vi "Self Configure.vi"(8 "error in (no error)":errorcluster, 11 "Instruments in":refnum<class "Instruments.lvclass">) -> (0 "error out":errorcluster, 3 "Instruments out":refnum<class "Instruments.lvclass">)   [LabVIEW 2023, in "Instruments.lvlib" / "Instruments.lvclass"]
uses:
  Library/Instruments.lvclass
  Custom Controls/Configuration Keys.ctl
  Library/Instruments.lvclass/Instruments.ctl
  builds/Framework/Configuration.lvlibp/Library/Configuration.lvclass
  C:/Users/Public/Documents/Development/builds/Framework/Configuration.lvlibp/Library/Configuration.lvclass
panel:
  in  "Configuration Keys":T1
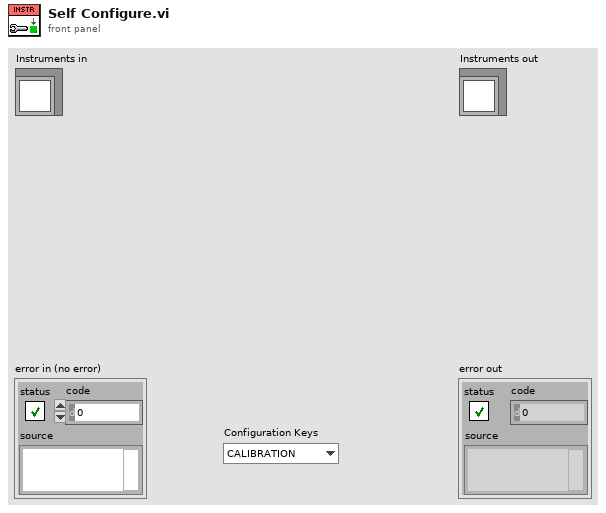
[diagram p1: front panel]
types:
  T1 = typedef "Instruments.lvlib/Instruments.lvclass/Configuration Keys.ctl" = enum16{"CALIBRATION", "RESOURCE", "POLL(MS)", "PANEL", "SIMULATED", "ENABLED"}
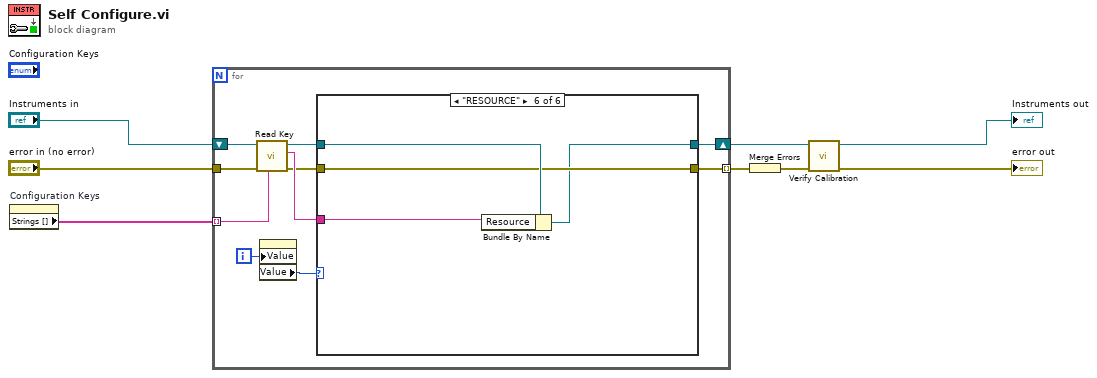
[diagram p0: block diagram]
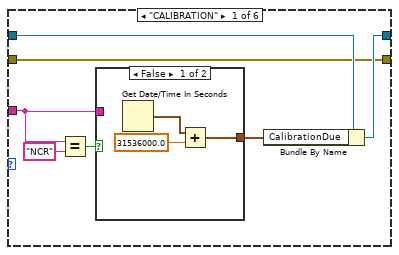
[diagram p2: hidden frame]
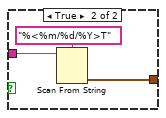
[diagram p3: hidden frame]
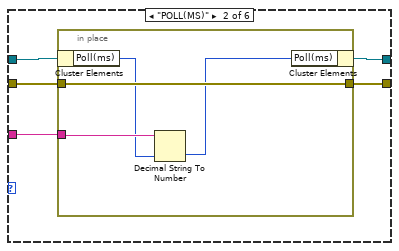
[diagram p4: hidden frame]
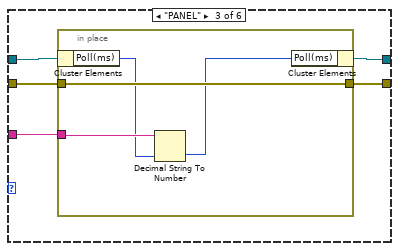
[diagram p5: hidden frame]
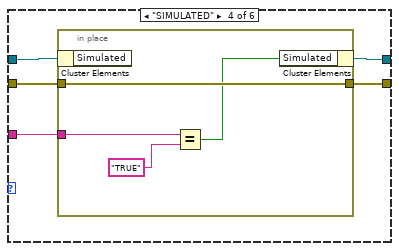
[diagram p6: hidden frame]
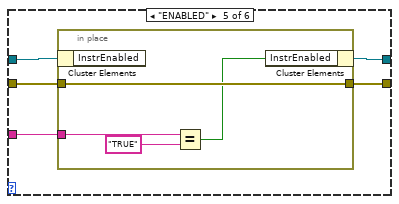
[diagram p7: hidden frame]
diagram:
  n1 = property on="Configuration Keys" class="Enum (strict)"() -> ("Strings []"=w7:string[])  [unwired: 2 in, 2 out]
  n2 = for {
    shift-right: [w10] -> w4
    shift-left: "Instruments in" -> [w16]
    tunnel: w7 -> [w13] mode=indexing
    tunnel: "error in (no error)" -> [w14]
    tunnel: [w9] -> w5 mode=indexing
    i -> [w18]
    n3 = call "Read Key.vi"("Key"=w13, "error in (no error)"=w14, "Configuration in"=w16) -> ("error out"=w11:errorcluster, "Value"=w12:string, "Configuration out"=w15:refnum<class "Instruments.lvclass">)  [unwired: 6 in]
    n4 = property on="Configuration Keys" class="Enum (strict)"("Value"=w18) -> ("Value"=w17:T1)  [unwired: 2 in, 2 out]
    n5 = case shown="\"RESOURCE\"" w17 {
      tunnel: w15 -> [w25 w36 w45 w54 w63 w71]
      tunnel: w12 -> [w19 w32 w41 w50 w59 w68]
      tunnel: w11 -> [w23 w34 w43 w52 w61 w70]
      tunnel: [w24 w35 w44 w53 w62 w69] -> w10
      tunnel: [w23 w33 w42 w51 w60 w70] -> w9
      frame "CALIBRATION" {
        n6 = Equal?(x=w19, y="NCR") -> (x = y?=w21:bool)
        n7 = case shown="False" w21 {
          tunnel: [w26 w29] -> w20
          tunnel: w19 -> [_ w31]
          frame False {
            n8 = Get Date/Time In Seconds() -> (seconds since 1Jan1904=w28:timestamp)
            n9 = Add(x=w28, y=31536000.0) -> (x+y=w26:timestamp)
          }
          frame True {
            n10 = Scan From String(format string="%<%m/%d/%Y>T", input string=w31) -> (output 1=w29:timestamp)  [unwired: 3 in, 3 out]
          }
        }
        n11 = Bundle By Name(cluster=w25, "CalibrationDue"=w20) -> (w24:refnum<class "Instruments.lvclass">)
      }
      frame "POLL(MS)" {
        n12 = in-place {
          in-place-border: w34 -> [w40]
          in-place-border: [w40] -> w33
          in-place-border: w32 -> [w39]
          n13 = in-place-cluster #1(w36) -> ("Poll(ms)"=w38:i32)
          n14 = Decimal String To Number(string=w39, default (0L)=w38) -> (number=w37:i32)  [unwired: 1 in, 1 out]
          n15 = in-place-cluster #1("Poll(ms)"=w37) -> (w35:refnum<class "Instruments.lvclass">)
        }
      }
      frame "PANEL" {
        n16 = in-place {
          in-place-border: w43 -> [w49]
          in-place-border: [w49] -> w42
          in-place-border: w41 -> [w48]
          n17 = in-place-cluster #2(w45) -> ("Poll(ms)"=w47:i32)
          n18 = Decimal String To Number(string=w48, default (0L)=w47) -> (number=w46:i32)  [unwired: 1 in, 1 out]
          n19 = in-place-cluster #2("Poll(ms)"=w46) -> (w44:refnum<class "Instruments.lvclass">)
        }
      }
      frame "SIMULATED" {
        n20 = in-place {
          in-place-border: w52 -> [w58]
          in-place-border: [w58] -> w51
          in-place-border: w50 -> [w57]
          n21 = in-place-cluster #3(w54) -> ()  [unwired: 1 out]
          n22 = Equal?(x=w57, y="TRUE") -> (x = y?=w55:bool)
          n23 = in-place-cluster #3("Simulated"=w55) -> (w53:refnum<class "Instruments.lvclass">)
        }
      }
      frame "ENABLED" {
        n24 = in-place {
          in-place-border: w61 -> [w67]
          in-place-border: [w67] -> w60
          in-place-border: w59 -> [w66]
          n25 = in-place-cluster #4(w63) -> ()  [unwired: 1 out]
          n26 = Equal?(x=w66, y="TRUE") -> (x = y?=w64:bool)
          n27 = in-place-cluster #4("InstrEnabled"=w64) -> (w62:refnum<class "Instruments.lvclass">)
        }
      }
      frame "RESOURCE" {
        n28 = Bundle By Name(cluster=w71, "Resource"=w68) -> (w69:refnum<class "Instruments.lvclass">)
      }
    }
  }
  n29 = Merge Errors(w5) -> (w3:errorcluster)
  n30 = call "Verify Calibration.vi"("error in"=w3, "Instruments in"=w4) -> ("error out"=→"error out":errorcluster, "Instruments out"=→"Instruments out":refnum<class "Instruments.lvclass">)  [unwired: 8 in]
